vi "To_More_Generic_Cluster.vi"(0 "Reference_In":refnum<vi>[](array[refnum])) -> (4 "Reference_Out":refnum<vi>[](array[refnum]))   [LabVIEW 2023]
doc: "Used to convert the reference to more generic."
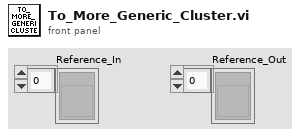
[diagram p1: front panel]
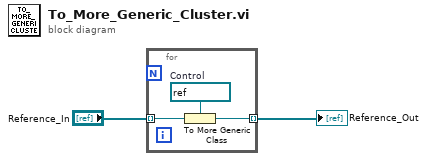
[diagram p0: block diagram]
diagram:
  n1 = for {
    tunnel: "Reference_In" -> [w5] mode=indexing
    tunnel: [w3] -> w2 mode=indexing
    w4 = refnum<vi> refnum  # Control
    n2 = To More Generic Class(target class=w4, reference=w5) -> (generic class reference=w3:refnum<vi>)
  }
  "Reference_Out" <- w2
